vi "ImageToArray.vi"(8 "error in (no error)":errorcluster, 11 "image":T1) -> (0 "error out":errorcluster, 1 "height":i32, 2 "width":i32, 3 "image data":sgl[](array[numeric]))   [LabVIEW 2017]
uses:
  <vilib>/vision/Image Controls.llb/IMAQ Image.ctl
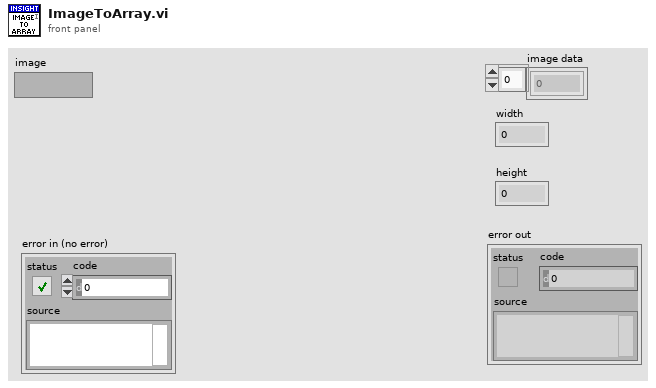
[diagram p1: front panel]
types:
  T1 = typedef "IMAQ Image.ctl" = refnum<image>
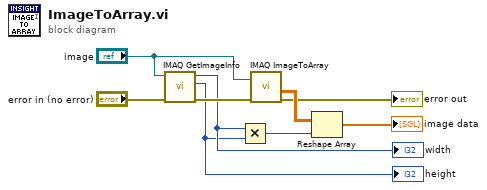
[diagram p0: block diagram]
diagram:
  n1 = call "IMAQ GetImageInfo"("error in (no error)"="error in (no error)", "Image"="image") -> ("error out"=w9:errorcluster, "Y Resolution"=w1:i32, "X Resolution"=w2:i32)  [unwired: 2 in, 5 out]
  "width" <- w2
  "height" <- w1
  n2 = Multiply(x=w2, y=w1) -> (x*y=w7:i32)
  n3 = call "IMAQ ImageToArray"("error in (no error)"=w9, "Image"="image") -> ("Image Pixels (Float)"=w8:sgl[][], "error out"=→"error out":errorcluster)  [unwired: 2 in, 3 out]
  n4 = Reshape Array(w8, w7) -> (→"image data":sgl[])
